vi "Generation of code word using msg and generator matri(SubVI).vi"(6 "G in":dbl[][](array[numeric]), 9 "messages in":i16[][](array[numeric]), 10 "n":i32, 11 "k":i32) -> (3 "Array":i32[][](array[numeric]))   [LabVIEW 2014]
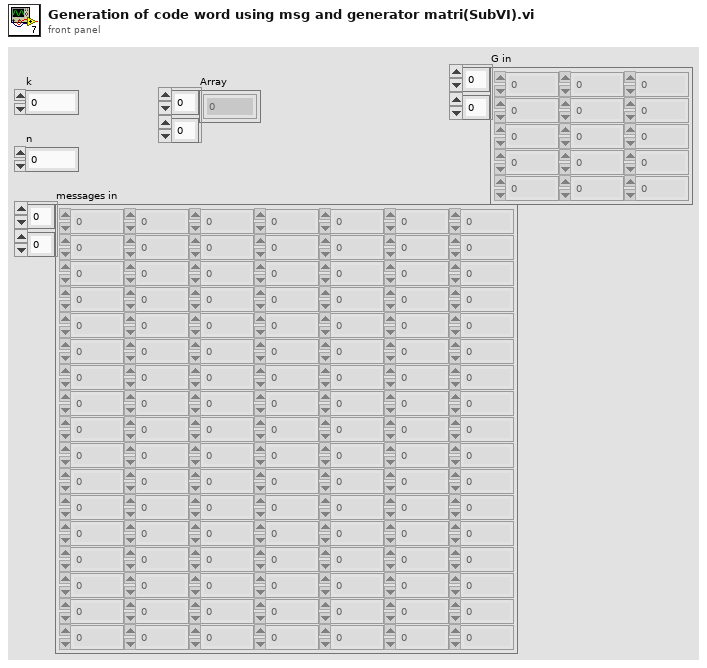
[diagram p1: front panel]
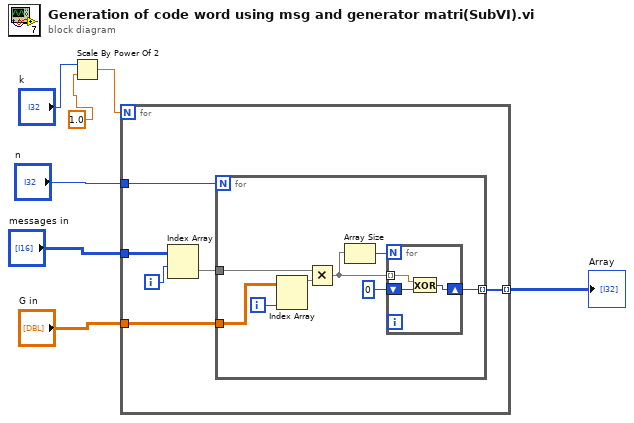
[diagram p0: block diagram]
diagram:
  n1 = Scale By Power Of 2(n="k", x=1.0) -> (x*2^n=w2:dbl)
  n2 = for {
    N: w2 -> [_]
    tunnel: "messages in" -> [w13]
    tunnel: "G in" -> [w12]
    tunnel: "n" -> [w10]
    tunnel: [w9] -> w3 mode=indexing
    i -> [w8]
    n3 = Index Array(array=w13, index (row)=w8) -> (element=w11:i16[])  [unwired: 1 in]
    n4 = for {
      N: w10 -> [_]
      tunnel: w12 -> [w21]
      tunnel: w11 -> [w19]
      tunnel: [w14] -> w9 mode=indexing
      i -> [w15]
      n5 = Index Array(array=w21, index (col)=w15) -> (element=w18:dbl[])  [unwired: 1 in]
      n6 = Multiply(x=w19, y=w18) -> (x*y=w16:dbl[])
      n7 = Array Size(array=w16) -> (size(s)=w17:i32)
      n8 = for {
        N: w17 -> [_]
        tunnel: w16 -> [w22] mode=indexing
        shift-right: [w23] -> w14
        shift-left: 0 -> [w24]
        n9 = Exclusive Or(1:w24, 2:w22) -> (0:w23:i32)
      }
    }
  }
  "Array" <- w3
